vi "SelectTrajectory.vi"() -> (3 "Robot Action Array":T1[](array[typedef]))   [LabVIEW 2018]
uses:
  Controls/Enable Actions.ctl
  Controls/Grip Motor Commands.ctl
  Controls/Lift Motor Commands.ctl
  Controls/Dics Eject Command.ctl
  Controls/Ball Motor Commands.ctl
  Controls/Arm Motor Commands.ctl
  Controls/Climb Motor Commands.ctl
  Controls/Pivot Motor Commands.ctl
  Controls/Robot Drive Mode.ctl
  Controls/Robot Pivot Motion Commands.ctl
  Controls/Robot State.ctl
  Controls/Robot Actions.ctl
panel:
  in  "Tab Control":enum32{"Climb Up", "Climb Down", "Page 3"}(tab)
  in  "Climb Up":T1[](array[typedef])
  # "Note that the first element in the trajectory is only the starting state and the duration is ignored."
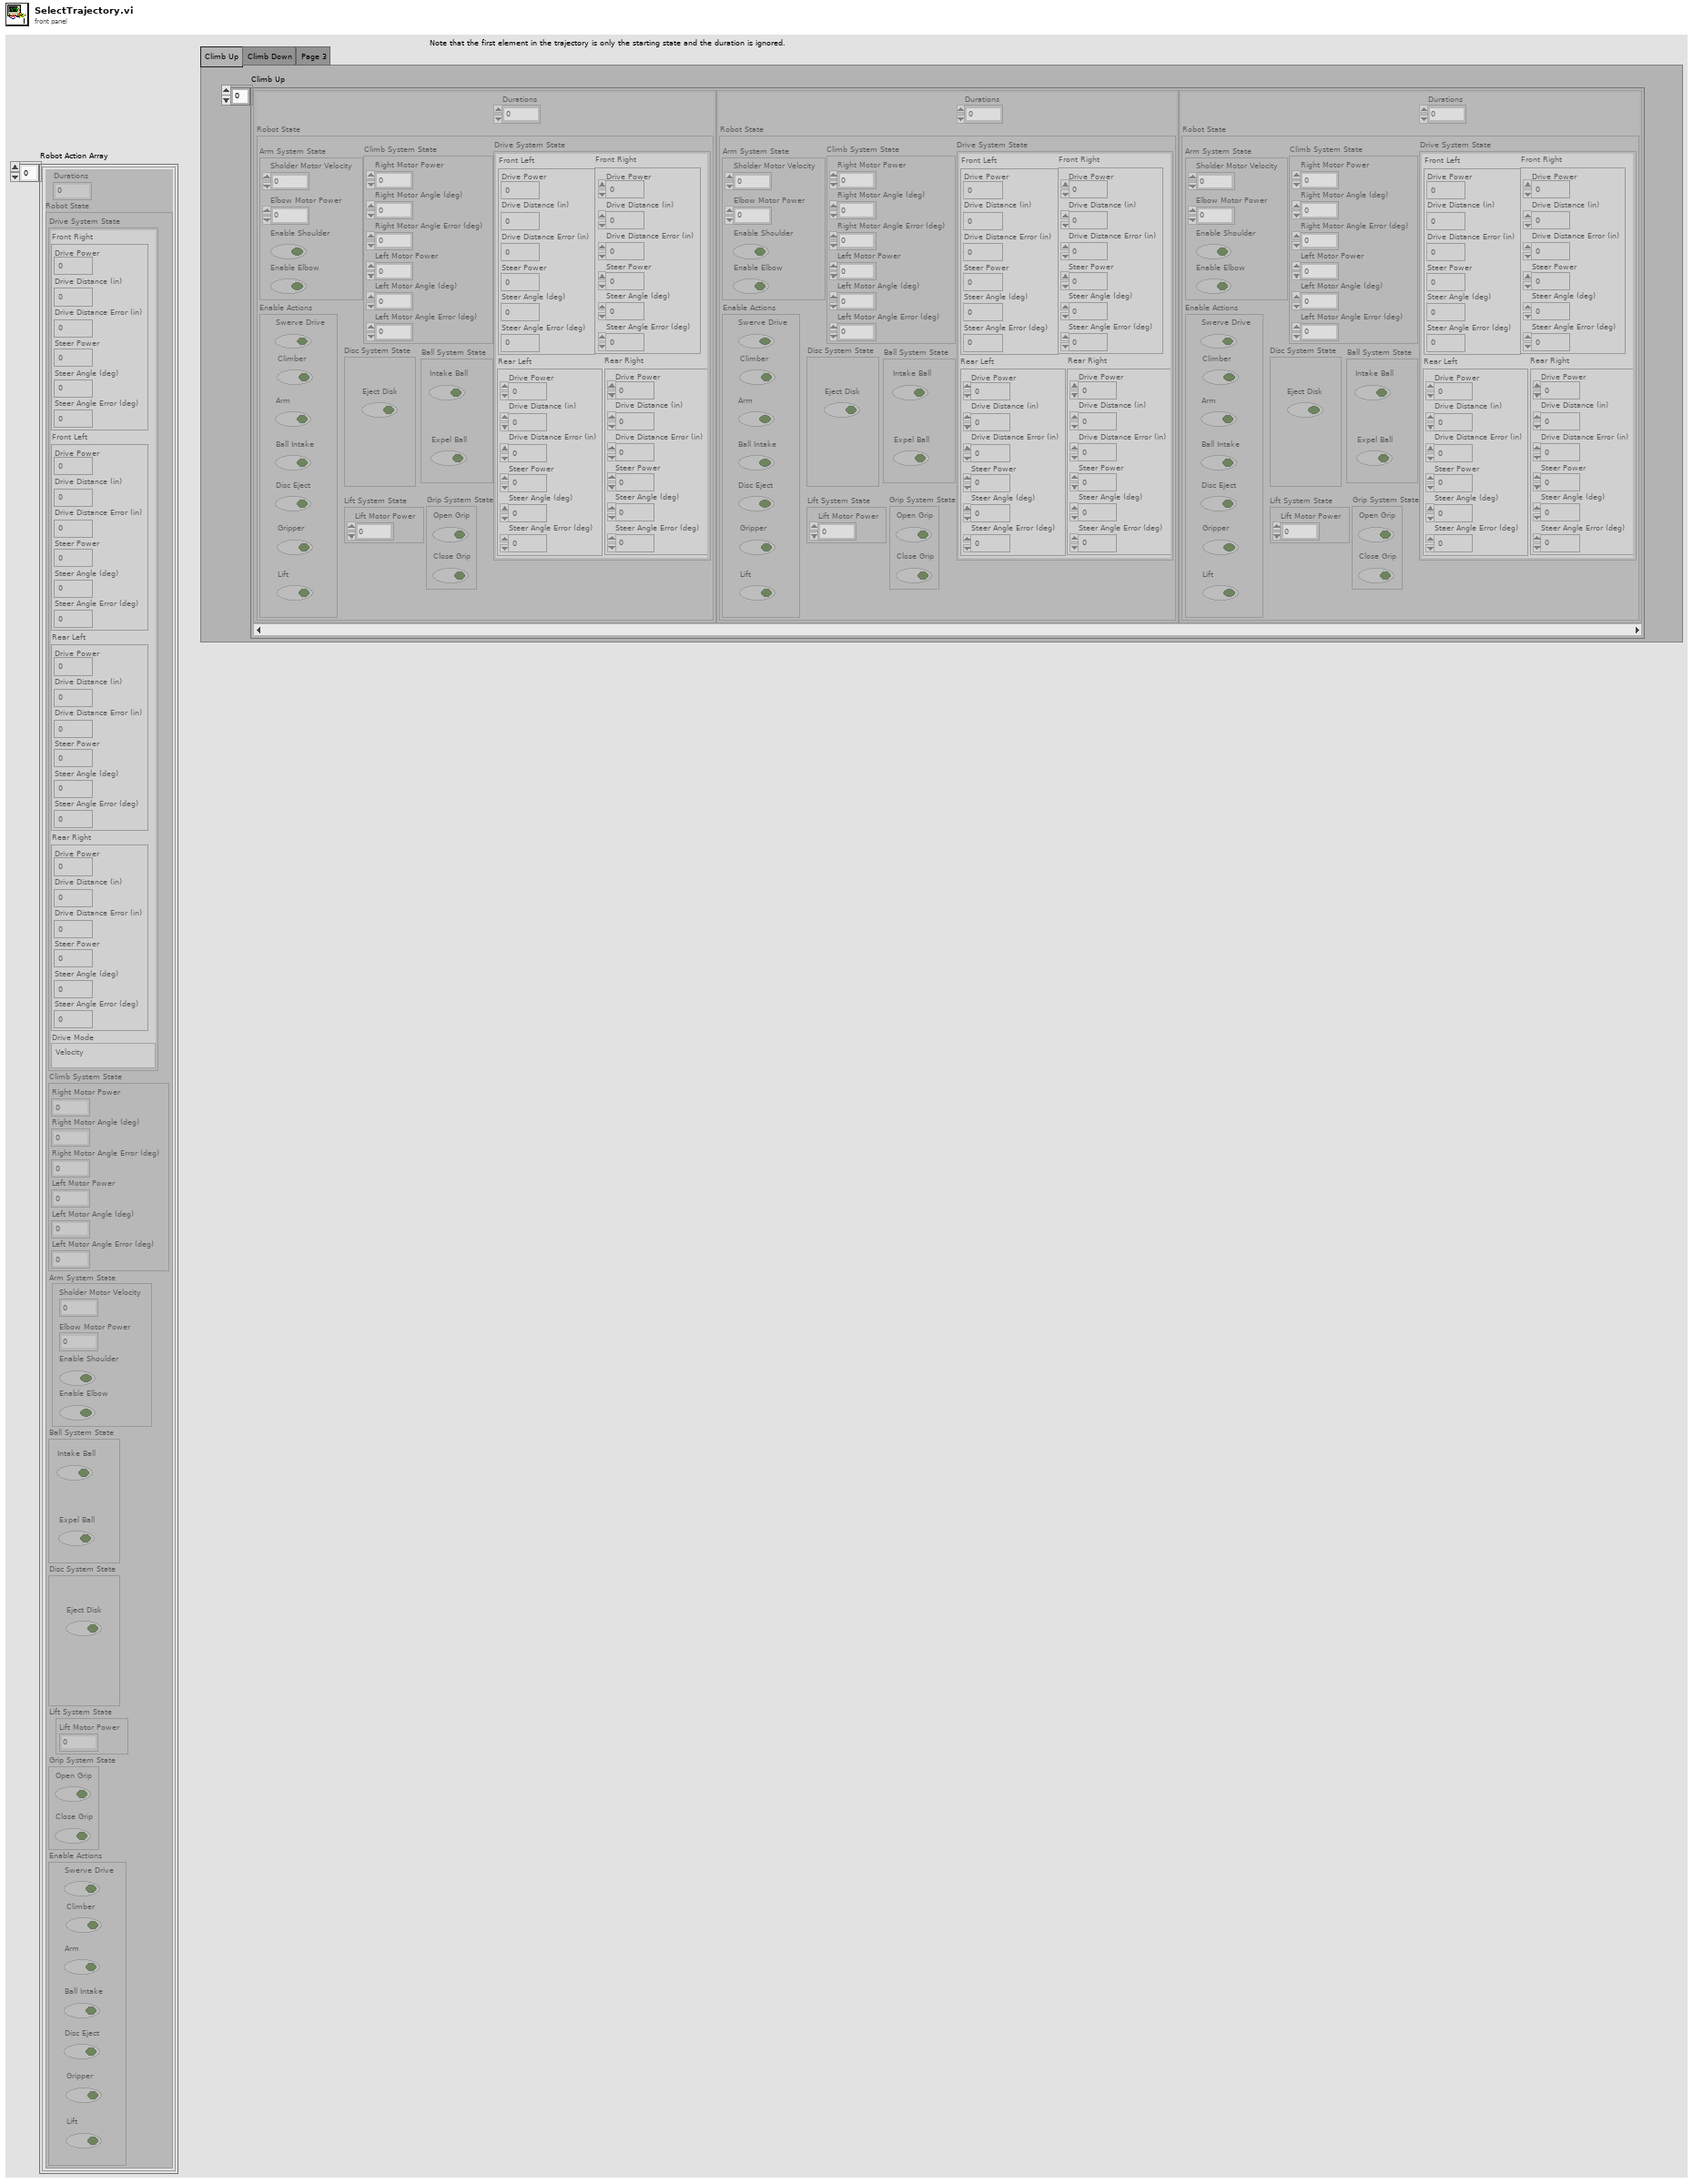
[diagram p1: front panel]
types:
  T1 = typedef "Robot Actions.ctl" = cluster{"Durations":dbl, "Robot State":T2}
  T2 = typedef "Robot State.ctl" = cluster{"Drive System State":T3, "Climb System State":T6, "Arm System State":T7, "Ball System State":T8, "Disc System State":T9, "Lift System State":T10, "Grip System State":T11, "Enable Actions":T12}
  T3 = typedef "Robot Pivot Motion Commands.ctl" = cluster{"Front Right":T4, "Front Left":T4, "Rear Left":T4, "Rear Right":T4, "Drive Mode":T5}
  T4 = typedef "Pivot Motor Commands.ctl" = cluster{"Drive Power":dbl, "Drive Distance (in)":dbl, "Drive Distance Error (in)":dbl, "Steer Power":dbl, "Steer Angle (deg)":dbl, "Steer Angle Error (deg)":dbl}
  T5 = typedef "Robot Drive Mode.ctl" = enum16{"Velocity", "Distance"}
  T6 = typedef "Climb Motor Commands.ctl" = cluster{"Right Motor Power":dbl, "Right Motor Angle (deg)":dbl, "Right Motor Angle Error (deg)":dbl, "Left Motor Power":dbl, "Left Motor Angle (deg)":dbl, "Left Motor Angle Error (deg)":dbl}
  T7 = typedef "Arm Motor Commands.ctl" = cluster{"Enable Shoulder":bool, "Enable Elbow":bool, "Elbow Motor Power":dbl, "Sholder Motor Velocity":dbl}
  T8 = typedef "Ball Motor Commands.ctl" = cluster{"Intake Ball":bool, "Expel Ball":bool}
  T9 = typedef "Dics Eject Command.ctl" = cluster{"Eject Disk":bool}
  T10 = typedef "Lift Motor Commands.ctl" = cluster{"Lift Motor Power":dbl}
  T11 = typedef "Grip Motor Commands.ctl" = cluster{"Open Grip":bool, "Close Grip":bool}
  T12 = typedef "Enable Actions.ctl" = cluster{"Swerve Drive":bool, "Climber":bool, "Arm":bool, "Ball Intake":bool, "Disc Eject":bool, "Gripper":bool, "Lift":bool}
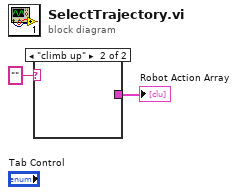
[diagram p0: block diagram]
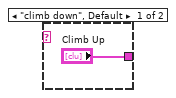
[diagram p2: hidden frame]
diagram:
  n1 = case shown="\"climb up\"" "" {
    tunnel: ["Climb Up" _] -> w1
    frame "climb down", Default {
    }
    frame "climb up" {
    }
  }
  "Robot Action Array" <- w1
